vi "Final Project.vi"() -> ()   [LabVIEW 2015]
uses:
  Temp monitor control.ctl
panel:
  in  "Numeric":i32=25
  out "Boolean 3":bool
  out "Boolean 2":bool
  out "Boolean":bool
  in  "Time Stamp Control":timestamp
  out "Temp Indicator alarm":string
  in  "Temp in F":bool
  out "Waveform Chart":cluster{dbl, dbl}(graph)
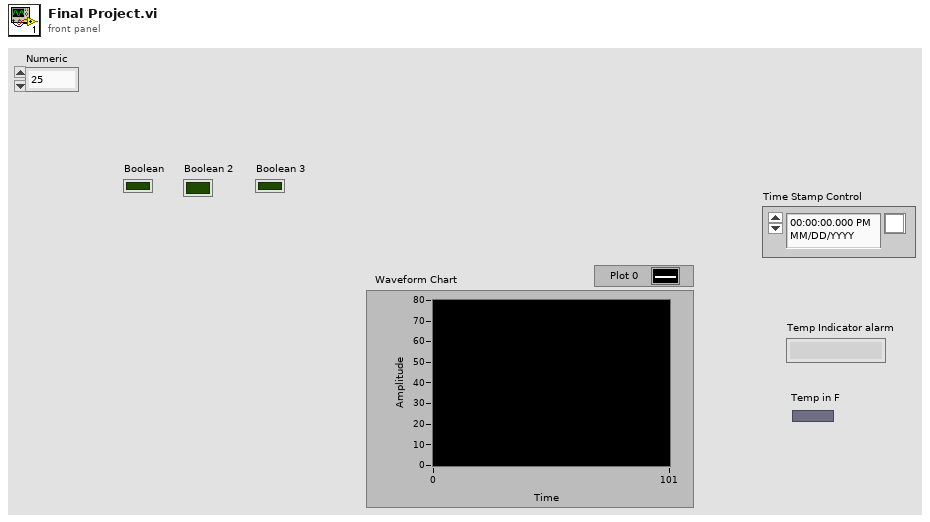
[diagram p1: front panel]
types:
  T1 = typedef "Temp monitor control.ctl" = enum16{"Start", "Temp Convertion", "T>25", "T>=60", "T>=75"}
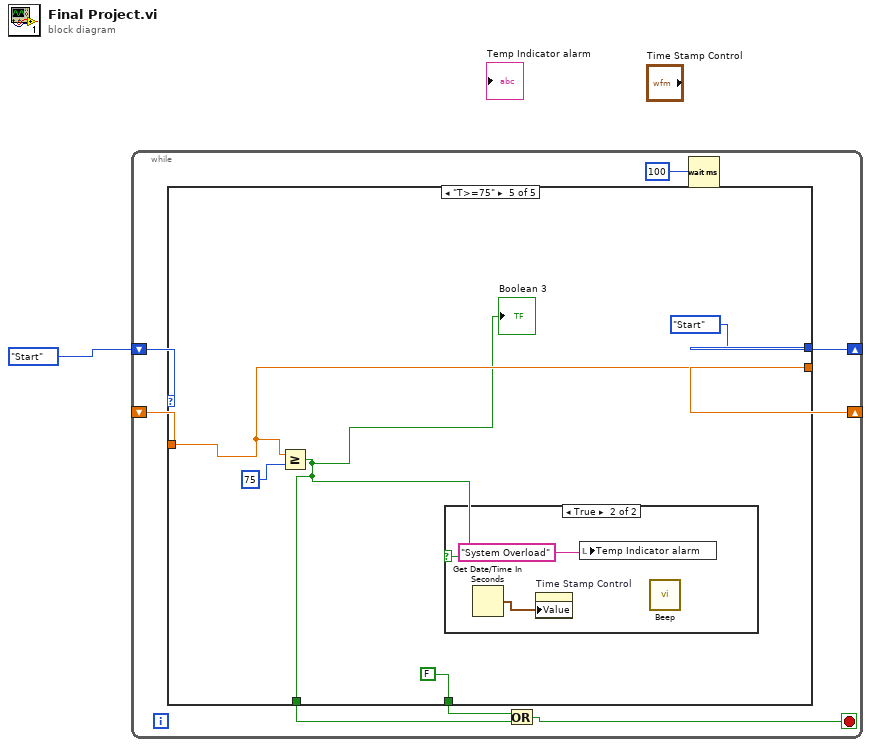
[diagram p0: block diagram]
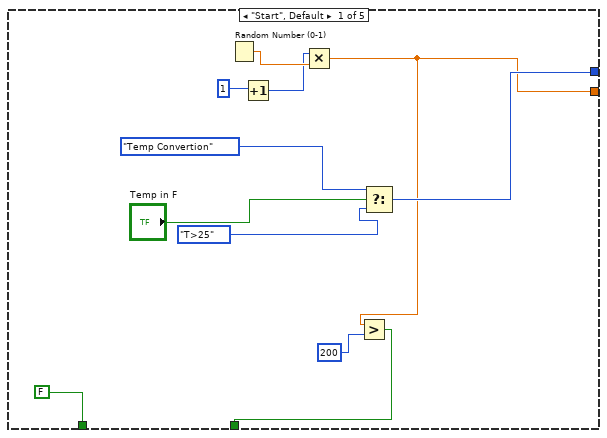
[diagram p2: hidden frame]
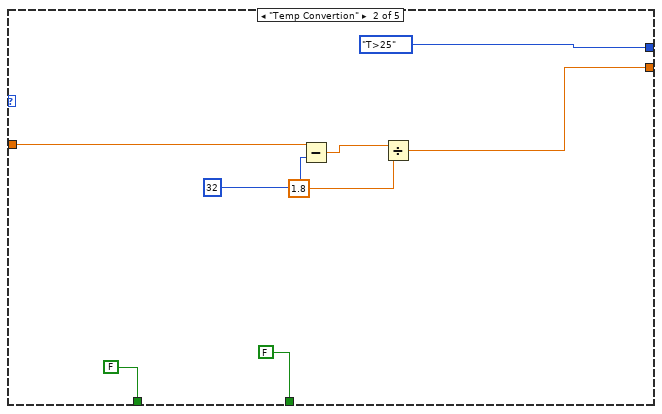
[diagram p3: hidden frame]
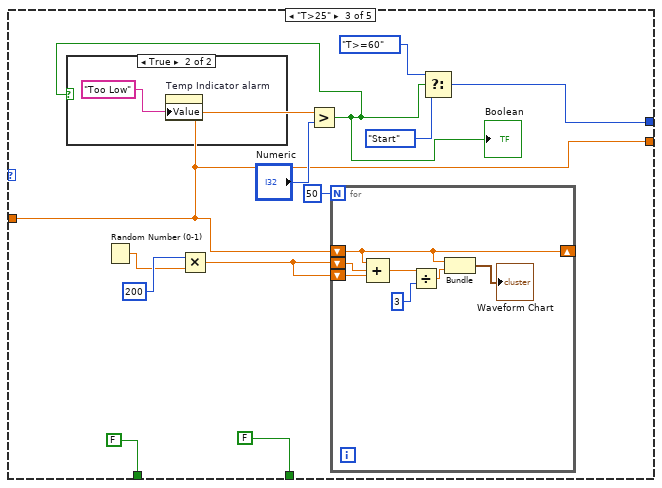
[diagram p4: hidden frame]
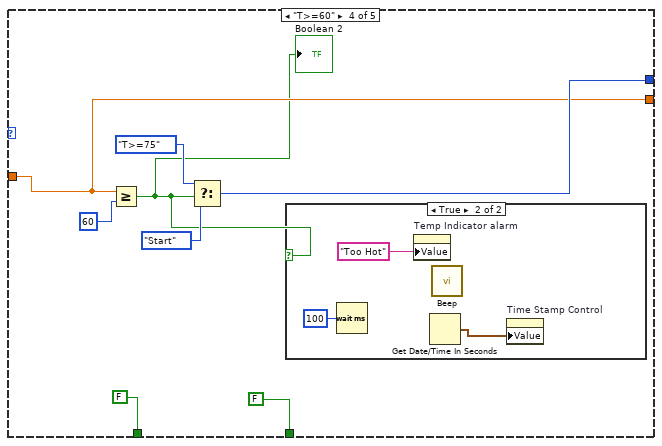
[diagram p6: hidden frame]
diagram:
  n1 = while {
    shift-right: [w7] -> _
    shift-left: Temp_monitor_control."Start" -> [w9]
    shift-right: [w8] -> _
    shift-left: _ -> [w6]
    stop <- w2 stop-if-true
    n2 = case shown="\"T>=75\"" w9 {
      tunnel: [w13 w24 w32 w52 w63] -> w8
      tunnel: w6 -> [_ w27 w32 w52 w63]
      tunnel: [w16 Temp_monitor_control."T>25" w37 w53 Temp_monitor_control."Start"] -> w7
      tunnel: [FALSE FALSE FALSE FALSE w62] -> w4
      tunnel: [w11 FALSE FALSE FALSE FALSE] -> w3
      frame "Start", Default {
        n3 = Random Number (0-1)() -> (number: 0 to 1=w20:dbl)
        n4 = Increment(x=1) -> (x+1=w14:i32)
        n5 = Multiply(x=w14, y=w20) -> (x*y=w13:dbl)
        n6 = Greater?(x=w13, y=200) -> (0:w11:bool)
        n7 = Select(t=Temp_monitor_control."Temp Convertion", s="Temp in F", f=Temp_monitor_control."T>25") -> (s? t:f=w16:T1)
      }
      frame "Temp Convertion" {
        n8 = Subtract(x=w27, y=32) -> (x-y=w25:dbl)
        n9 = Divide(x=w25, y=1.8) -> (x/y=w24:dbl)
      }
      frame "T>25" {
        n10 = Random Number (0-1)() -> (number: 0 to 1=w34:dbl)
        n11 = Multiply(x=200, y=w34) -> (x*y=w33:dbl)
        n12 = Greater?(x=w32, y="Numeric") -> (0:w30:bool)
        "Boolean" <- w30
        n13 = case shown="True" w30 {
          frame False {
          }
          frame True {
            n14 = property on="Temp Indicator alarm" class="Str"("Value"="Too Low" ("String")) -> ()  [unwired: 2 in, 2 out]
          }
        }
        n15 = for {
          N: 50 -> [_]
          shift-right: [w43] -> _
          shift-left: w32 -> [w43]
          shift-left: w33 -> [w48]
          shift-left: w33 -> [w47]
          n16 = Compound Arithmetic op=ADD(w43, w48, w47) -> (w46:dbl)
          n17 = Divide(x=w46, y=3) -> (x/y=w44:dbl)
          n18 = Bundle(w43, w44) -> (→"Waveform Chart":cluster{dbl, dbl})  [unwired: 1 in]
        }
        n19 = Select(t=Temp_monitor_control."T>=60", s=w30, f=Temp_monitor_control."Start") -> (s? t:f=w37:T1)
      }
      frame "T>=60" {
        n20 = Greater Or Equal?(x=w52, y=60) -> (x >= y?=w50:bool)
        "Boolean 2" <- w50
        n21 = Select(t=Temp_monitor_control."T>=75", s=w50, f=Temp_monitor_control."Start") -> (s? t:f=w53:T1)
        n22 = case shown="True" w50 {
          frame False {
          }
          frame True {
            n23 = Wait (ms)(milliseconds to wait=u32 100) -> ()  [unwired: 1 out]
            n24 = property on="Temp Indicator alarm" class="Str"("Value"="Too Hot") -> ()  [unwired: 2 in, 2 out]
            n25 = Get Date/Time In Seconds() -> (seconds since 1Jan1904=w57:timestamp)
            n26 = call <vilib>:"Beep.vi"() -> ()  [unwired: 12 in]
            n27 = property on="Time Stamp Control" class="AbsTime (strict)"("Value"=w57) -> ()  [unwired: 2 in, 2 out]
          }
        }
      }
      frame "T>=75" {
        n28 = Greater Or Equal?(x=w63, y=75) -> (x >= y?=w62:bool)
        "Boolean 3" <- w62
        n29 = case shown="True" w62 {
          frame False {
          }
          frame True {
            n30 = Get Date/Time In Seconds() -> (seconds since 1Jan1904=w66:timestamp)
            n31 = property on="Time Stamp Control" class="AbsTime (strict)"("Value"=w66) -> ()  [unwired: 2 in, 2 out]
            n32 = local write "Temp Indicator alarm"("System Overload") -> ()
            n33 = call <vilib>:"Beep.vi"() -> ()  [unwired: 12 in]
          }
        }
      }
    }
    n34 = Or(x=w3, y=w4) -> (x .or. y?=w2:bool)
    n35 = Wait (ms)(milliseconds to wait=u32 100 ("millisecond timer value")) -> ()  [unwired: 1 out]
  }
